vi "19.Evd.7_Ask.3.vi"() -> ()   [LabVIEW 2025]
panel:
  in  "stop":bool
  out "Result":string
  in  "Password":string
  in  "Username":string
  in  "Username - Password":string[][](array[string])
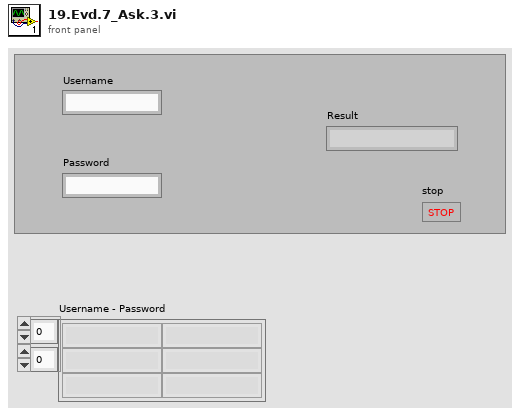
[diagram p1: front panel]
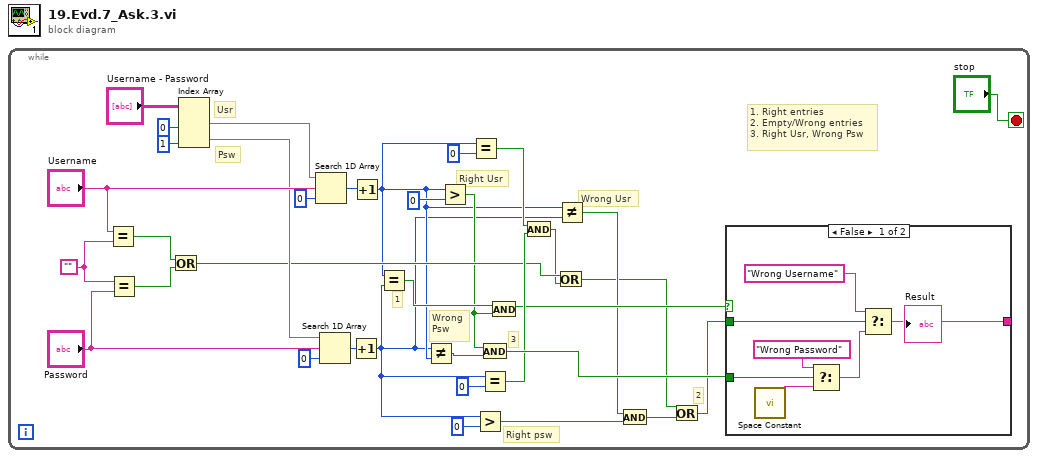
[diagram p0: block diagram]
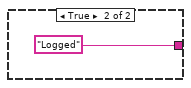
[diagram p2: hidden frame]
diagram:
  n1 = while {
    stop <- "stop" stop-if-true
    w32 = ""
    # "Wrong\nPsw"
    # "Right Usr"
    # "Wrong Usr"
    # "Right psw"
    # "3"
    # "2"
    # "1. Right entries\n2. Empty/Wrong entries\n3. Right Usr, Wrong Psw"
    # "1"
    # "Psw"
    # "Usr"
    n2 = Equal?(x="Username", y=w32) -> (x = y?=w31:bool)
    n3 = Equal?(x=w32, y="Password") -> (x = y?=w30:bool)
    n4 = Or(x=w31, y=w30) -> (x .or. y?=w13:bool)
    n5 = Index Array(array="Username - Password", index (col) #1=0 ("disabled index (col)"), index (col) #2=1 ("index (col)")) -> (element #1=w28:string[], element #2=w24:string[])  [unwired: 2 in]
    n6 = Search 1D Array(1D array=w28, element="Username", start index (0)=0) -> (index of element=w26:i32)
    n7 = Search 1D Array(1D array=w24, element="Password", start index (0)=0) -> (index of element=w21:i32)
    n8 = Increment(x=w21) -> (x+1=w5:i32)
    n9 = Increment(x=w26) -> (x+1=w6:i32)
    n10 = Equal?(x=w6, y=w5) -> (x = y?=w11:bool)
    n11 = Not Equal?(x=w5, y=w6) -> (x != y?=w18:bool)
    n12 = Greater?(x=w6, y=0) -> (0:w10:bool)
    n13 = Equal?(x=w6, y=0) -> (x = y?=w15:bool)
    n14 = Greater?(x=w5, y=0) -> (0:w7:bool)
    n15 = And(x=w10, y=w18) -> (x .and. y?=w19:bool)
    n16 = Equal?(x=w5, y=0) -> (x = y?=w14:bool)
    n17 = And(x=w11, y=w10) -> (x .and. y?=w9:bool)
    n18 = And(x=w15, y=w14) -> (x .and. y?=w12:bool)
    n19 = Or(x=w13, y=w12) -> (x .or. y?=w2:bool)
    n20 = Not Equal?(x=w6, y=w5) -> (x != y?=w4:bool)
    n21 = And(x=w4, y=w7) -> (x .and. y?=w1:bool)
    n22 = Or(x=w2, y=w1) -> (x .or. y?=w3:bool)
    n23 = case shown="False" w9 {
      tunnel: [w41 "Logged"] -> w20
      tunnel: w3 -> [w43 _]
      tunnel: w19 -> [w40 _]
      frame False {
        n24 = call <vilib>:"Space Constant.vi"() -> ("String"=w37:string)
        n25 = Select(t="Wrong Password", s=w40, f=w37) -> (s? t:f=w38:string)
        n26 = Select(t="Wrong Username", s=w43, f=w38) -> (s? t:f=w41:string)
      }
      frame True {
      }
    }
    "Result" <- w20
  }
